vi "Stabilize_Bath.vi"() -> ()   [LabVIEW 2019]
uses:
  Monitors/Utility/Monitor Communication/LS370/LS370-Control.ctl
  Global/Global Variables/Data_Display_global.vi
  Instrument_Setup.vi
  Monitors/Utility/Monitor Communication/sub-vis/LS370_Open_Queue.vi
panel:
  out "MC-Bath offset":dbl
  out "MC setpoint reached":bool
  out "MC current":dbl
  out "MC Setpoint":dbl
  out "Bath current":dbl
  in  "Bath Target":dbl
  out "Tolerance (%)":dbl
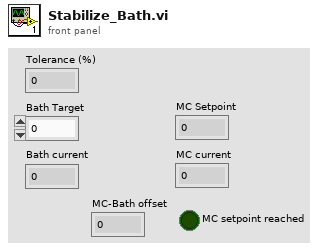
[diagram p1: front panel]
types:
  T1 = typedef "LS370_Status.ctl" = cluster{"Setpoint":dbl, "MC Heater Output":dbl, "Still Heater Output":dbl, "Sorb  Heater Output":dbl, "LS370 T1":dbl, "LS370 T2":dbl, "LS370 T3":dbl, "LS370 T4":dbl, "LS370 T5":dbl, "LS370 R1":dbl, "LS370 R2":dbl, "LS370 R3":dbl, "LS370 R4":dbl, "LS370 R5":dbl, "LS370 T6":dbl, "LS370 T7":dbl, "LS370 T8":dbl, "LS370 T9":dbl, "LS370 R6":dbl, "LS370 R7":dbl, "LS370 R8":dbl, "LS370 R9":dbl, "LS370 TC-T":dbl, "LS370 TC-R":dbl}
  T2 = typedef "LS372_read_only-Cluster.ctl" = cluster{"LS372-T1":dbl, "LS372 -T2":dbl, "LS372-T4":dbl, "LS372-T5":dbl, "LS372-T6":dbl, "LS372-R1 ":dbl, "LS372-R2":dbl, "LS372-R3 ":dbl, "LS372-R4 \n\n\n\n":dbl, "LS372-R5":dbl, "LS372-R6 ":dbl, "LS372-T3":dbl, "Update Lakeshores":bool}
  T3 = typedef "LS370-Control.ctl" = cluster{"Disable Heater":bool, "Activate Tsweep":bool, "Update Lakeshores":bool, "Setpoint - Manual":dbl, "Rate (K/min)":dbl, "Sorb Power (mW)":dbl, "Still Power (mW)":dbl, "Sorb Heater":bool, "Still Heater":bool, "Set Temperature Sweep Main":bool}
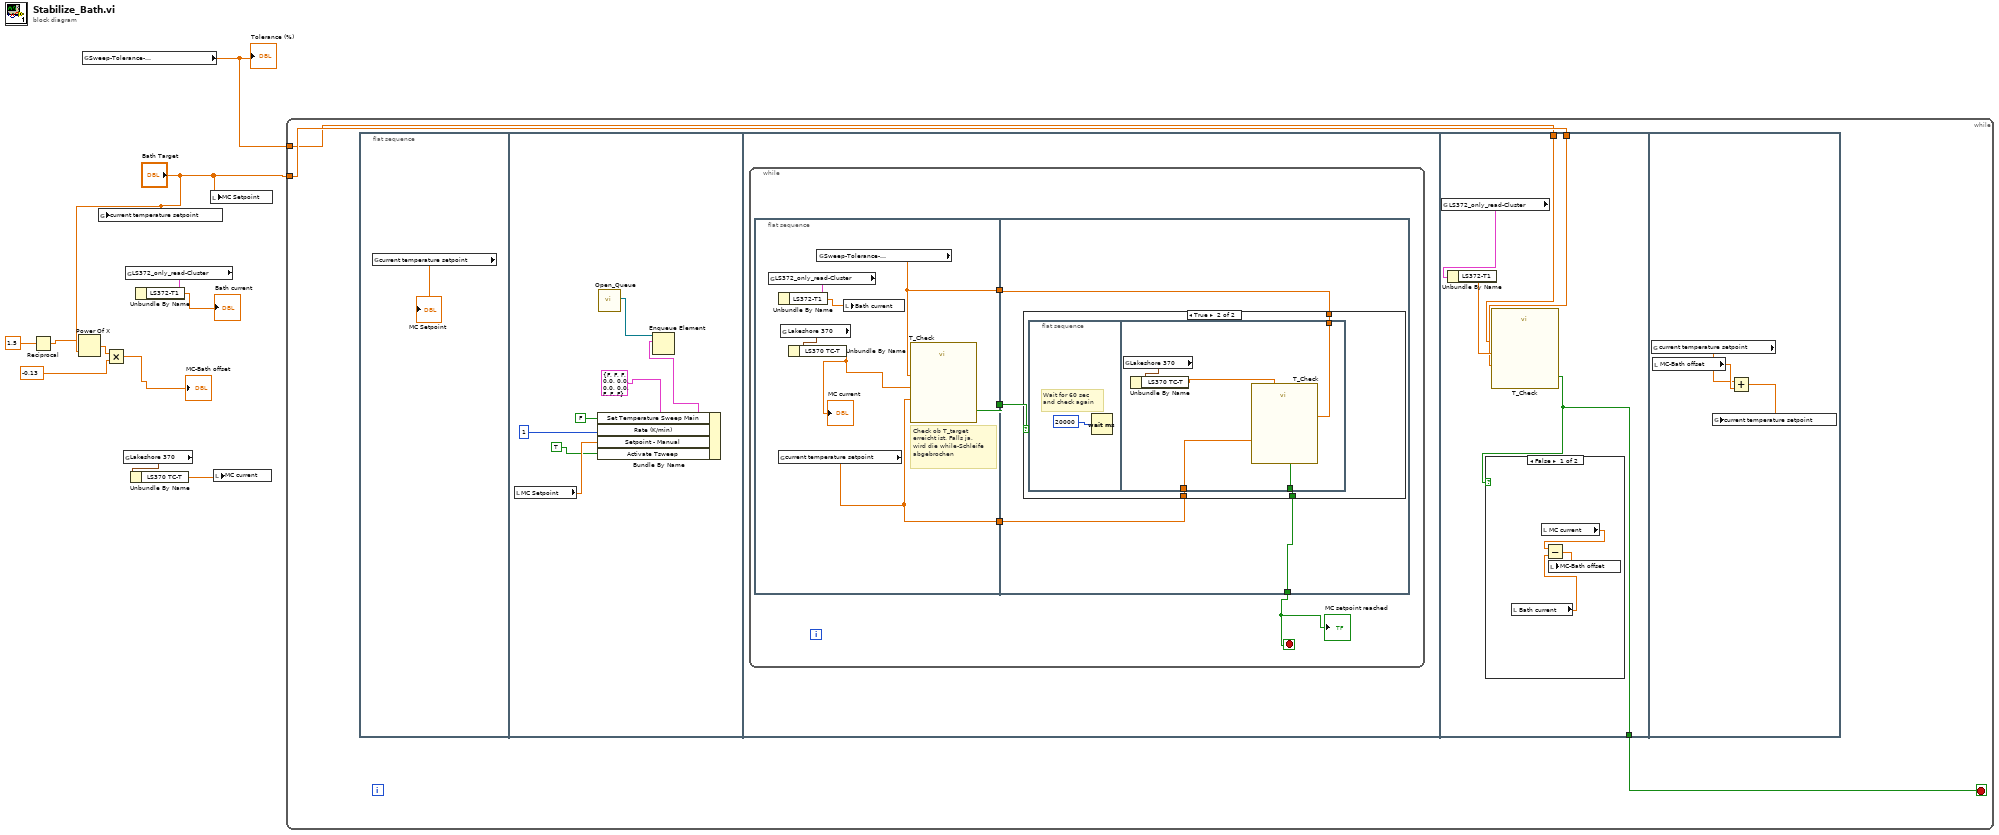
[diagram p0: block diagram]
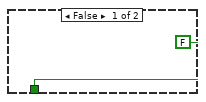
[diagram p2: hidden frame]
diagram:
  n1 = Reciprocal(x=1.5) -> (1/x=w4:dbl)
  n2 = Power Of X(1:"Bath Target", 2:w4) -> (0:w3:dbl)
  n3 = global read "Instrument_Setup.vi" "Sweep-Tolerance-\nTemperature"() -> (w9:dbl)
  "Tolerance (%)" <- w9
  n4 = global write "Data_Display_global.vi" "current temperature setpoint"("Bath Target") -> ()
  n5 = Multiply(x=w3, y=-0.13) -> (x*y=→"MC-Bath offset":dbl)
  n6 = global read "Data_Display_global.vi" "Lakeshore 370"() -> (w8:T1)
  n7 = global read "Data_Display_global.vi" "LS372_only_read-Cluster"() -> (w11:T2)
  n8 = Unbundle By Name(w8) -> ("LS370 TC-T"=w7:dbl)
  n9 = Unbundle By Name(w11) -> ("LS372-T1"=→"Bath current":dbl)
  n10 = local write "MC Setpoint"("Bath Target") -> ()
  n11 = local write "MC current"(w7) -> ()
  n12 = while {
    tunnel: "Bath Target" -> [w13]
    tunnel: w9 -> [w12]
    stop <- w14 stop-if-true
    n13 = flat-sequence {
      tunnel: [w50] -> w14
      tunnel: w13 -> [w49]
      tunnel: w12 -> [w48]
      frame #0 {
        n14 = global read "Data_Display_global.vi" "current temperature setpoint"() -> (→"MC Setpoint":dbl)
      }
      frame #1 {
        n15 = local read "MC Setpoint"() -> (w18:dbl)
        n16 = Bundle By Name(cluster=T3 {"Disable Heater"=FALSE, "Activate Tsweep"=FALSE, "Update Lakeshores"=FALSE, "Setpoint - Manual"=0.0, "Rate (K/min)"=0.0, "Sorb Power (mW)"=0.0, "Still Power (mW)"=0.0, "Sorb Heater"=FALSE, "Still Heater"=FALSE, "Set Temperature Sweep Main"=FALSE} ("JT-Cluster"), "Set Temperature Sweep Main"=FALSE, "Rate (K/min)"=1, "Setpoint - Manual"=w18, "Activate Tsweep"=TRUE) -> (w19:T3)
        n17 = call-poly "Open_Queue.vi"() -> ("queue out"=w22:refnum<queue>)  [unwired: 10 in, 1 out]
        n18 = Enqueue Element(queue=w22, element=w19) -> ()  [unwired: 2 in, 3 out]
      }
      frame #2 {
        n19 = while {
          stop <- w23 stop-if-true
          n20 = flat-sequence {
            tunnel: [w33] -> w26
            tunnel: [w31] -> w25
            tunnel: [w32] -> w24
            tunnel: w26 -> [w37]
            tunnel: w25 -> [w36]
            tunnel: w24 -> [w35]
            tunnel: [w34] -> w23
            frame #0 {
              # "Check ob T_target\nerreicht ist. Falls ja,\nwird die while-Schleife\nabgebrochen"
              n21 = global read "Data_Display_global.vi" "LS372_only_read-Cluster"() -> (w28:T2)
              n22 = Unbundle By Name(w28) -> ("LS372-T1"=w27:dbl)
              n23 = global read "Data_Display_global.vi" "current temperature setpoint"() -> (w31:dbl)
              n24 = global read "Data_Display_global.vi" "Lakeshore 370"() -> (w30:T1)
              n25 = Unbundle By Name(w30) -> ("LS370 TC-T"=w29:dbl)
              "MC current" <- w29
              n26 = global read "Instrument_Setup.vi" "Sweep-Tolerance-\nTemperature"() -> (w32:dbl)
              n27 = local write "Bath current"(w27) -> ()
              n28 = call "T_Check.vi"("Sweep\nTolerance %"=w32, "T_target (K)"=w31, "T_in"=w29) -> ("= T target"=w33:bool)
            }
            frame #1 {
              n29 = case shown="True" w37 {
                tunnel: w36 -> [_ w41]
                tunnel: w35 -> [_ w40]
                tunnel: [FALSE w39] -> w34
                frame False {
                }
                frame True {
                  n30 = flat-sequence {
                    tunnel: w41 -> [w47]
                    tunnel: w40 -> [w46]
                    tunnel: [w45] -> w39
                    frame #0 {
                      # "Wait for 60 sec\nand check again"
                      n31 = Wait (ms)(milliseconds to wait=20000) -> ()  [unwired: 1 out]
                    }
                    frame #1 {
                      n32 = global read "Data_Display_global.vi" "Lakeshore 370"() -> (w44:T1)
                      n33 = Unbundle By Name(w44) -> ("LS370 TC-T"=w43:dbl)
                      n34 = call "T_Check.vi"("Sweep\nTolerance %"=w46, "T_target (K)"=w47, "T_in"=w43) -> ("= T target"=w45:bool)
                    }
                  }
                }
              }
            }
          }
          "MC setpoint reached" <- w23
        }
      }
      frame #3 {
        n35 = global read "Data_Display_global.vi" "LS372_only_read-Cluster"() -> (w51:T2)
        n36 = Unbundle By Name(w51) -> ("LS372-T1"=w52:dbl)
        n37 = call "T_Check.vi"("Sweep\nTolerance %"=w48, "T_target (K)"=w49, "T_in"=w52) -> ("= T target"=w50:bool)
        n38 = case shown="False" w50 {
          frame False {
            n39 = local read "Bath current"() -> (w53:dbl)
            n40 = local read "MC current"() -> (w54:dbl)
            n41 = Subtract(x=w54, y=w53) -> (x-y=w55:dbl)
            n42 = local write "MC-Bath offset"(w55) -> ()
          }
          frame True {
          }
        }
      }
      frame #4 {
        n43 = global read "Data_Display_global.vi" "current temperature setpoint"() -> (w56:dbl)
        n44 = local read "MC-Bath offset"() -> (w57:dbl)
        n45 = Add(x=w56, y=w57) -> (x+y=w58:dbl)
        n46 = global write "Data_Display_global.vi" "current temperature setpoint"(w58) -> ()
      }
    }
  }
